vi "KE622x -- Set Buf Num Readings For Notify.vi"(0 "Resource In":refnum<visa-resource-name>, 1 "Check For SCPI Errors? (T)":bool=TRUE, 7 "Num Reads For Notify":T1=1 min=1 max=65535 step=1, 11 "error in (no error)":errorcluster) -> (4 "Resource Out (dupl)":refnum<visa-resource-name>, 15 "error out":errorcluster)   [LabVIEW 2009, in "Keithley 622x.lvlib"]
uses:
  Keithley 622x.lvlib
  Typedefs/KE622x -- Trace Buf Num Reads For Notify.ctl
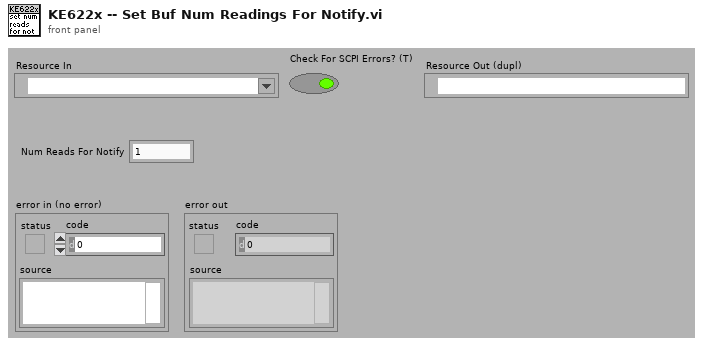
[diagram p1: front panel]
types:
  T1 = typedef "Keithley 622x.lvlib/KE622x -- Trace Buf Num Reads For Notify.ctl" = u32
  T2 = typedef "Keithley 622x.lvlib/KE622x -- Trace Buf Size.ctl" = u32
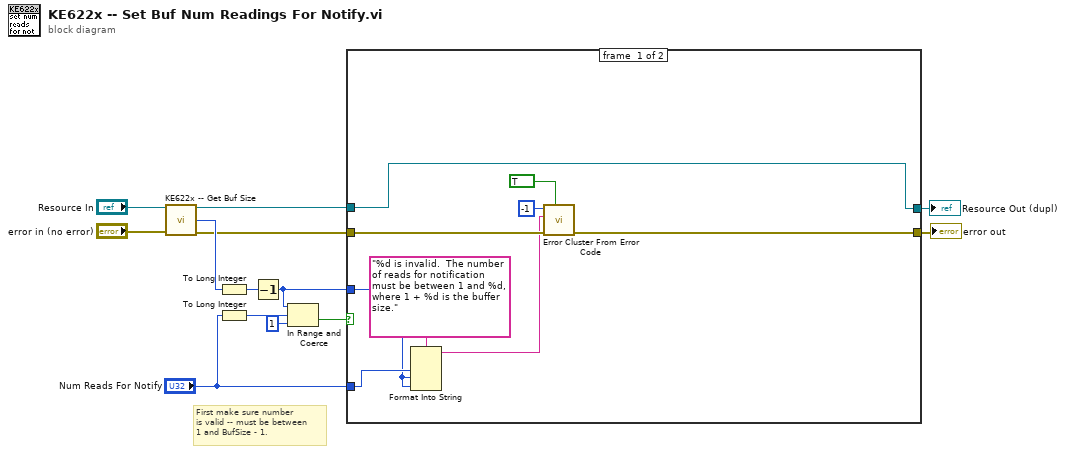
[diagram p0: block diagram]
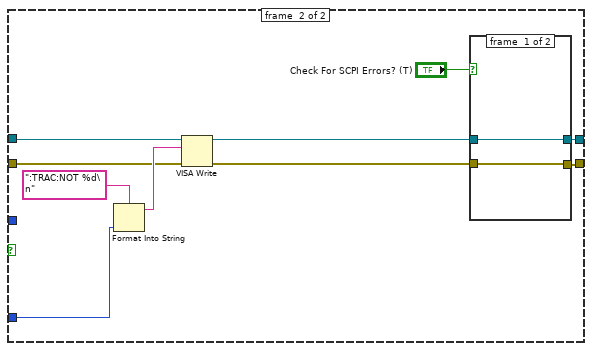
[diagram p2: hidden frame]
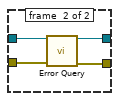
[diagram p3: hidden frame]
diagram:
  # "First make sure number\nis valid -- must be between\n1 and BufSize - 1."
  n1 = call "KE622x -- Get Buf Size.vi"("Resource In"="Resource In", "error in (no error)"="error in (no error)") -> ("Resource Out (dupl)"=w1:refnum<visa-resource-name>, "Buffer Size (Num Readings)"=w9:T2, "error out"=w2:errorcluster)  [unwired: 11 in]
  n2 = To Long Integer(number=w9) -> (32bit integer=w8:i32)
  n3 = To Long Integer(number="Num Reads For Notify") -> (32bit integer=w7:i32)
  n4 = Decrement(x=w8) -> (x-1=w4:i32)
  n5 = In Range and Coerce(upper limit=w4, x=w7, lower limit=1) -> (In Range?=w5:bool)  [unwired: 1 out]
  n6 = case shown="True" w5 {
    tunnel: [w15 w28] -> w13
    tunnel: [w14 w27] -> w12
    tunnel: w4 -> [w20 _]
    tunnel: "Num Reads For Notify" -> [w21 w23]
    tunnel: w2 -> [w19 w25]
    tunnel: w1 -> [w15 w26]
    frame #0 {
      n7 = Format Into String(format string="%d is invalid.  The number of reads for notification must be between 1 and %d, where 1 + %d is the buffer size.", w21, w20, w20) -> (resulting string=w18:string)  [unwired: 2 in, 1 out]
      n8 = call <vilib>:"Error Cluster From Error Code.vi"("show call chain? (False)"=TRUE, "error in (no error)"=w19, "error message (\"\")"=w18, "error code (0)"=-1) -> ("error out"=w14:errorcluster)  [unwired: 5 in]
    }
    frame #1 {
      n9 = Format Into String(format string=":TRAC:NOT %d\n", w23) -> (resulting string=w31:string)  [unwired: 2 in, 1 out]
      n10 = VISA Write(VISA resource name=w26, write buffer=w31, error in (no error)=w25) -> (VISA resource name out=w30:refnum<visa-resource-name>, error out=w29:errorcluster)  [unwired: 1 out]
      n11 = case shown="True" "Check For SCPI Errors? (T)" {
        tunnel: w30 -> [w34 w38]
        tunnel: w29 -> [w33 w37]
        tunnel: [w33 w36] -> w27
        tunnel: [w34 w35] -> w28
        frame #0 {
        }
        frame #1 {
          n12 = call "Error Query.vi"("VISA Resource In"=w38, "error in (no error)"=w37) -> ("VISA Resource Out (dupl)"=w35:refnum<visa-resource-name>, "error out"=w36:errorcluster)  [unwired: 10 in, 2 out]
        }
      }
    }
  }
  "Resource Out (dupl)" <- w13
  "error out" <- w12
